vi "Obtain Table Buffer.vi"(7 "Buffer Size (10k)":i32=10000 format="%.0p", 8 "error in (no error)":errorcluster, 9 "Create (F)":bool) -> (0 "error out":errorcluster, 3 "Table Queue":refnum<queue>)   [LabVIEW 2025, in "I2C Bus Monitor UI.lvlib"]
uses:
  I2C Bus Monitor UI.lvlib
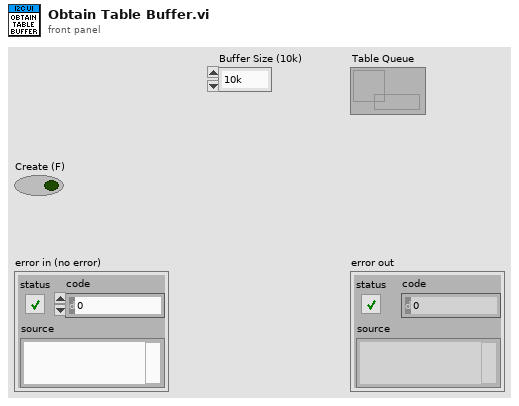
[diagram p1: front panel]
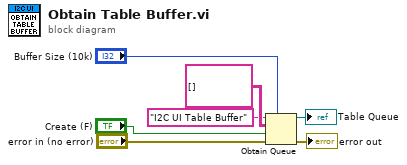
[diagram p0: block diagram]
diagram:
  n1 = Obtain Queue(max queue size (-1, unlimited)="Buffer Size (10k)", name (unnamed)="I2C UI Table Buffer", element data type=string[][] [] ("I2C Messages"), create if not found? (T)="Create (F)", error in (no error)="error in (no error)") -> (queue out=→"Table Queue":refnum<queue>, error out=→"error out":errorcluster)  [unwired: 1 out]
